vi "HFRR ADV v015 new software.vi"() -> ()   [LabVIEW 2025] (continued)
                n4021 = Subtract(x=w5264, y=w5269) -> (x-y=w5268:u32)
                n4022 = Select(t=w5268, s=w5267, f=u32 0) -> (s? t:f=w5265:u32)
                n4023 = while {
                  tunnel: w5270 -> [w5303]
                  tunnel: [w5305] -> w5263 mode=indexing
                  tunnel: w5265 -> [w5287]
                  i -> [w5304]
                  stop <- w5302 stop-if-true
                  w5294 = 6 ("index")
                  w5293 = 2 ("length")
                  # "Page 65 of \nmanual"
                  n4024 = Multiply(x=u32 3 ("y"), y=w5304) -> (x*y=w5301:u32)
                  n4025 = Divide(x=u32 102 ("y"), y=u32 65520) -> (x/y=w5311:dbl)
                  n4026 = Greater Or Equal?(x=w5301, y=w5287) -> (x >= y?=w5302:bool)
                  n4027 = Index Array(array=w5303, index (row) #1=w5301) -> (element #1=w5299:bool[], element #2=w5298:bool[], element #3=w5297:bool[])  [unwired: 5 in]
                  n4028 = Reverse 1D Array(array=w5299) -> (reversed array=w5292:bool[])
                  n4029 = Reverse 1D Array(array=w5298) -> (reversed array=w5296:bool[])
                  n4030 = Reverse 1D Array(array=w5297) -> (reversed array=w5295:bool[])
                  n4031 = Delete From Array(array=w5292, length=w5293, index=w5294) -> (array with subset deleted=w5288:bool[])  [unwired: 1 out]
                  n4032 = Delete From Array(array=w5296, length=w5293, index=w5294) -> (array with subset deleted=w5289:bool[])  [unwired: 1 out]
                  n4033 = Delete From Array(array=w5295, length=w5293, index=w5294) -> (array with subset deleted=w5290:bool[])  [unwired: 1 out]
                  n4034 = Insert Into Array(array=bool[] [] ("Boolean array"), new element #1=w5288, new element #2=w5289, new element #3=w5290) -> (w5291:bool[])  [unwired: 1 in]
                  n4035 = Boolean Array To Number(Boolean array=w5291) -> (number=w5300:u32)
                  n4036 = Multiply(x=w5311, y=w5300) -> (x*y=w5310:dbl)
                  n4037 = Decrement(x=w5310) -> (x-1=w5309:dbl)
                  n4038 = Divide(x=w5309, y=u32 100) -> (x/y=w5307:dbl)
                  n4039 = Multiply(x=w5307, y=u32 10) -> (x*y=w5305:dbl)
                }
                n4040 = Delete From Array(array=w5263) -> (array with subset deleted=w5262:dbl[])  [unwired: 2 in, 1 out]
                "Waveform Graph 5" <- w5262
                "Waveform Chart 3" <- w5262
                n4041 = call-poly <vilib>:"Mean.vi"("X"=w5262) -> ("mean"=w5261:dbl)  [unwired: 1 out]
                n4042 = case shown="True" {
                  selector: _ -> [_ _]
                  tunnel: w5261 -> [_ w5286]
                  frame False {
                  }
                  frame True {
                    n4043 = local write item#-1(FALSE ("Zero 4")) -> ()
                    "z_measure" <- w5286
                  }
                }
              }
            }
            n4044 = local read item#-1() -> (w5201)
            n4045 = local read item#-1() -> (w5200)
            n4046 = local read item#-1() -> (w5202)
            n4047 = local read item#-1() -> (w5199)
            n4048 = case shown="True" w5197 {
              tunnel: w5201 -> [_ w5229]
              tunnel: w5202 -> [_ w5228]
              frame False {
              }
              frame True {
                n4049 = Build Array(w5229, w5228) -> (w5227:void[])
                n4050 = local read item#-1() -> (w5232)
                n4051 = Build Array (concatenate)(w5232, w5227) -> (w5230:void[])
                n4052 = local write item#-1(w5230) -> ()
                n4053 = local write item#-1(FALSE ("Boolean 8")) -> ()
              }
            }
            n4054 = call "Build XY Graph"("Enable"=w5199, "Reset"=w5200, "Y Input"=w5202, "X Input"=w5201) -> ("XY Graph"=w5198:cluster{"Y":dbl[], "Y":dbl[]}[])  [unwired: 6 in, 1 out]
            n4055 = case shown="True" {
              selector: _ -> [_ _]
              frame False {
              }
              frame True {
                n4056 = local read item#-1() -> (w5233)
                n4057 = Index Array(array=w5233, index (col) #1=0 ("disabled index (col)"), index (col) #2=1 ("index (col)")) -> (element #1=w5235, element #2=w5234)  [unwired: 2 in]
                n4058 = call <vilib>:"Linear Fit.vi"("Y"=w5235, "X"=w5234) -> ()  [unwired: 9 in, 5 out]
                n4059 = local write item#-1(FALSE ("Boolean 9")) -> ()
              }
            }
            n4060 = case shown="True" {
              selector: _ -> [_ _]
              frame False {
              }
              frame True {
                n4061 = local write item#-1(dbl[][] [] ("Captured Values")) -> ()
                n4062 = local write item#-1(FALSE ("Boolean 7")) -> ()
              }
            }
            n4063 = Concatenate Strings("\r", "\n") -> (w5212:string, w5211:string)
            n4064 = case shown="True" w5203 {
              tunnel: w5210 -> [w5242 w5248]
              tunnel: w5209 -> [w5241 w5247]
              tunnel: [w5242 w5246] -> w5208
              tunnel: [w5241 w5245] -> w5207
              tunnel: w5212 -> [_ w5244]
              frame False {
              }
              frame True {
                n4065 = VISA Write(VISA resource name=w5248, write buffer=w5244, error in (no error)=w5247) -> (VISA resource name out=w5246:refnum<visa-resource-name>, error out=w5245:errorcluster)  [unwired: 1 out]
                n4066 = local write item#-1(FALSE ("WRITE")) -> ()
              }
            }
          }
          frame Error {
            w5336 = u16 10 items=["1.0"=10, "1.5"=15, "2.0"=20] ("stop bits (10: 1 bit)")
            n4067 = Wait (ms)(milliseconds to wait=u32 20) -> ()  [unwired: 1 out]
            n4068 = VISA Close(VISA resource name=w5338, error in (no error)=w5344) -> (error out=w5343:errorcluster)
            n4069 = call <vilib>:"Clear Errors.vi"("error in (no error)"=w5343) -> ("error out"=w5342:errorcluster)  [unwired: 5 in, 1 out]
            n4070 = call-poly "VISA Configure Serial Port"("timeout (10sec)"=u32 200, "Enable Termination\nChar (T)"=TRUE ("Enable Termination\nChar (T)"), "baud rate (9600)"=u32 921600, "error in (no error)"=w5342, "stop bits (10: 1 bit)"=w5336) -> ("VISA resource name"=w5334:refnum<visa-resource-name>, "VISA resource name out"=w5346:refnum<visa-resource-name>, "error out"=w5345:errorcluster)  [unwired: 8 in]
          }
        }
        n4071 = local read "Quit"() -> (w5186:bool)
      }
      n4072 = VISA Close(VISA resource name=w5181, error in (no error)=w5182) -> (error out=w5180:errorcluster)
      n4073 = call <vilib>:"Clear Errors.vi"("error in (no error)"=w5180) -> ()  [unwired: 5 in, 2 out]
    }
    frame Enabled {
    }
  }
  n4074 = disable-structure shown="Disabled" {
    disable-tunnel: _ -> [w5351 _]
    frame Disabled {
      n4075 = while {
        tunnel: [w5358] -> _
        shift-right: [w5355] -> w5348
        shift-left: _ -> [w5357]
        shift-right: [w5356] -> w5349
        shift-left: errorcluster {"status"=TRUE, "code"=0, "source"="Init"} ("error out") -> [w5354]
        tunnel: w5351 -> [_]
        i -> [w5358]
        stop <- w5352 stop-if-true
        n4076 = flat-sequence {
          tunnel: w5354 -> [w5449]
          tunnel: [w5449] -> w5353
          frame #0 {
            n4077 = Wait (ms)(milliseconds to wait=u32 50) -> ()  [unwired: 1 out]
          }
        }
        n4078 = case shown="No Error" w5353 {
          selector: w5353 -> [w5399 w5442]
          tunnel: w5357 -> [w5398 w5441]
          tunnel: [w5365 w5432] -> w5356
          tunnel: [w5366 w5440] -> w5355
          frame No Error {
            w5392 = T33 {"Mode"=enum."RTU", "Slave Address"=1} ("Serial Parameters")
            n4079 = call-poly <vilib>:"MB Serial Master Query (poly).vi"("VISA resource name"=w5398, "Starting Address"=i16 1000, "Quantity"=u16 1, "Timeout"=u32 1000, "error in"=w5399, "Serial Parameters"=w5392) -> ("VISA resource name out"=w5393:refnum<visa-resource-name>, "Input Registers"=w5395:u16[], "error out"=w5391:errorcluster)  [unwired: 10 in, 1 out]
            n4080 = Random Number (0-1)() -> (number: 0 to 1=w5380:dbl)
            n4081 = Index Array(array=w5395, index=0) -> (element=w5390:u16)
            n4082 = Subtract(x=w5380, y=0.5) -> (x-y=w5379:dbl)
            n4083 = Divide(x=w5390, y=10 ("index")) -> (x/y=w5384:dbl)
            n4084 = Multiply(x=w5379, y=0.5) -> (x*y=w5378:dbl)
            n4085 = Add(x=w5384, y=w5378) -> (x+y=w5383:dbl)
            n4086 = local read "Amb temp"() -> (w5367:dbl)
            n4087 = Multiply(x=w5383, y=0.2) -> (x*y=w5387:dbl)
            n4088 = Multiply(x=w5367, y=0.8) -> (x*y=w5385:dbl)
            n4089 = Add(x=w5387, y=w5385) -> (x+y=w5368:dbl)
            n4090 = local read "set temp old"() -> (w5362:dbl)
            n4091 = local write "Amb temp"(w5368) -> ()
            n4092 = Select(t="SetTemp 2", s="Heater", f=100.0) -> (s? t:f=w5363:dbl)
            n4093 = Not Equal?(x=w5363, y=w5362) -> (x != y?=w5361:bool)
            n4094 = case shown="True" w5361 {
              tunnel: w5393 -> [w5427 w5429]
              tunnel: [w5426 w5429] -> w5373
              tunnel: w5391 -> [w5425 w5428]
              tunnel: [w5424 w5428] -> w5371
              tunnel: w5363 -> [w5419 _]
              tunnel: w5392 -> [w5421 w5430]
              tunnel: [w5421 w5430] -> w5374
              frame True {
                n4095 = Multiply(x=w5419, y=10 ("index")) -> (x*y=w5418:dbl)
                n4096 = call-poly <vilib>:"MB Serial Master Query (poly).vi"("VISA resource name"=w5427, "Address"=u16 0, "Holding Register"=w5418, "Timeout"=u32 1000, "error in"=w5425, "Serial Parameters"=w5421) -> ("VISA resource name out"=w5426:refnum<visa-resource-name>, "error out"=w5424:errorcluster)  [unwired: 11 in, 1 out]
                "set temp old" <- w5419
              }
              frame False {
              }
            }
            n4097 = flat-sequence {
              tunnel: [w5400] -> _
              tunnel: [w5400] -> w5370
              tunnel: w5371 -> [w5400]
              frame #0 {
                n4098 = Wait (ms)(milliseconds to wait=u32 100) -> ()  [unwired: 1 out]
              }
            }
            n4099 = call "Elapsed Time12"("Time Target (s)"=2.0, "Auto Reset"=TRUE) -> ("Time has Elapsed"=w5375:bool)  [unwired: 10 in, 7 out]
            n4100 = case shown="True" w5375 {
              tunnel: w5374 -> [w5404 w5417]
              tunnel: [w5404 w5417] -> _
              tunnel: [w5403 w5415] -> w5366
              tunnel: w5373 -> [w5403 w5416]
              tunnel: [w5402 w5413] -> w5365
              tunnel: w5370 -> [w5402 w5414]
              frame False {
              }
              frame True {
                n4101 = call-poly <vilib>:"MB Serial Master Query (poly).vi"("VISA resource name"=w5416, "Starting Address"=i16 1003 ("Addr"), "Quantity"=u16 1, "Timeout"=u32 1000, "error in"=w5414, "Serial Parameters"=w5417) -> ("VISA resource name out"=w5415:refnum<visa-resource-name>, "Input Registers"=w5410:u16[], "error out"=w5413:errorcluster)  [unwired: 10 in, 1 out]
                n4102 = Index Array(array=w5410, index=0) -> (element=w5409:u16)
                n4103 = Divide(x=w5409, y=u16 10) -> (x/y=w5405:dbl)
                n4104 = local write "set temp old"(w5405) -> ()
                n4105 = local write "SetTemp"(w5405) -> ()
              }
            }
            "Error Code" <- w5365
            n4106 = Unbundle(w5365) -> ("status"=→"TK4 status":bool)  [unwired: 2 out]
            "SetTemp" <- "SetTemp 2"
          }
          frame Error {
            w5444 = u16 0 items=["None", "Odd", "Even", "Mark", "Space"] ("Parity")
            w5445 = u16 0 items=["None", "XON/XOFF", "RTS/CTS", "XON/XOFF & RTS/CTS", "DTR/DSR", "XON/XOFF & DTR/DSR"] ("Flow Control")
            n4107 = VISA Clear(VISA resource name=w5441, error in (no error)=w5442) -> (VISA resource name out=w5435:refnum<visa-resource-name>, error out=w5433:errorcluster)
            n4108 = VISA Close(VISA resource name=w5435, error in (no error)=w5433) -> (error out=w5434:errorcluster)
            n4109 = call <vilib>:"Clear Errors.vi"("error in (no error)"=w5434) -> ("error out"=w5443:errorcluster)  [unwired: 5 in, 1 out]
            n4110 = Unbundle By Name(T33 {"Mode"=enum."RTU", "Slave Address"=1} ("input cluster")) -> ("Mode"=w5446:enum16{"RTU", "ASCII"})
            n4111 = call <vilib>:"MB Serial Init.vi"("Timeout"=u32 100, "Flow Control"=w5445, "Mode"=w5446, "error in (no error)"=w5443, "Parity"=w5444, "Baud Rate"=u32 9600, "VISA resource name"="Lubrication System COM Port :") -> ("error out"=w5432:errorcluster, "VISA resource name out"=w5440:refnum<visa-resource-name>)  [unwired: 3 in]
            n4112 = local write "set temp old"(0.0 ("set temp old")) -> ()
            n4113 = Unbundle(w5432) -> ("status"=w5431:bool)  [unwired: 2 out]
            n4114 = case shown="True" w5431 {
              selector: w5431 -> [_ w5448]
              frame False {
              }
              frame True {
                n4115 = local write "TK4 status"(w5448) -> ()
              }
            }
          }
        }
        n4116 = local read "Quit"() -> (w5352:bool)
      }
      n4117 = VISA Close(VISA resource name=w5348, error in (no error)=w5349) -> (error out=w5347:errorcluster)
      n4118 = call <vilib>:"Clear Errors.vi"("error in (no error)"=w5347) -> ()  [unwired: 5 in, 2 out]
    }
    frame Enabled {
    }
  }
